vi "Shooter Mode Selector.vi"(9 "Set To Manual?":bool, 10 "Set To Safe?":bool, 11 "Set To Auto?":bool) -> (3 "Mode":T1)   [LabVIEW 2015]
uses:
  Common Code/Shoot Modes Enum.ctl
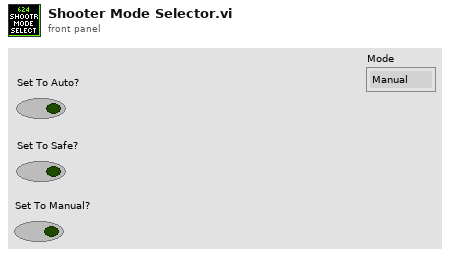
[diagram p1: front panel]
types:
  T1 = typedef "Shoot Modes Enum.ctl" = enum16{"Manual", "Safe", "Auto"}
  T2 = enum16{"0", "1", "2", "3", "4", "5", "6", "7", "8", "9", "A", "B", "C", "D", "E", "F", "G", "H", "I", "J", "K", "L", "M", "N", "O", "P", "Q", "R", "S", "T", "U", "V", "W", "X", "Y", "Z", "F1", "F2", "F3", "F4", "F5", "F6", "F7", "F8", "F9", "F10", "F11", "F12", "F13", "F14", "F15", "ADD", "BACK", "BACKSLASH", "CAPITAL", "COMMA", "DECIMAL", "DELETE", "DIVIDE", "DOWN", "END", "EQUALS", "ESCAPE", "GRAVE (`)", "HOME", "INSERT", "LBRACKET", "LCONTROL", "LEFT", "L ALT", "LSHIFT", "LWIN", "MINUS", "MULTIPLY", "NEXT", "NUMLOCK", "NUMPAD_0", "NUMPAD_1", "NUMPAD_2", "NUMPAD_3", "NUMPAD_4", "NUMPAD_5", "NUMPAD_6", "NUMPAD_7", "NUMPAD_8", "NUMPAD_9", "PAUSE", "PERIOD", "PRIOR (PG UP)", "RBRACKET", "RCONTROL", "RETURN", "RIGHT", "R ALT", "RSHIFT", "RWIN", "SCROLL", "SEMICOLON", "SLASH", "SPACE", "SUBTRACT", "TAB", "UP", "ENTER (num pad)", "' (quote)"}
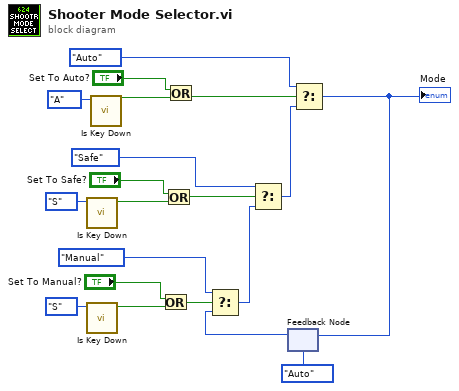
[diagram p0: block diagram]
diagram:
  n1 = call "Is Key Down.vi"("Key"=T2."S") -> ("Key Down?"=w14:bool)  [unwired: 10 in]
  n2 = call "Is Key Down.vi"("Key"=T2."S") -> ("Key Down?"=w10:bool)  [unwired: 10 in]
  n3 = call "Is Key Down.vi"("Key"=T2."A") -> ("Key Down?"=w19:bool)  [unwired: 10 in]
  n4 = Or(x="Set To Manual?", y=w10) -> (x .or. y?=w9:bool)
  n5 = Or(x="Set To Safe?", y=w14) -> (x .or. y?=w13:bool)
  n6 = Or(x="Set To Auto?", y=w19) -> (x .or. y?=w17:bool)
  n7 = feedback #1(Shoot_Modes_Enum."Auto" ("Mode")) -> (w2:T1)
  n8 = Select(t=Shoot_Modes_Enum."Manual" ("Mode"), s=w9, f=w2) -> (s? t:f=w4:T1)
  n9 = Select(t=Shoot_Modes_Enum."Safe" ("Mode"), s=w13, f=w4) -> (s? t:f=w5:T1)
  n10 = Select(t=Shoot_Modes_Enum."Auto" ("Mode"), s=w17, f=w5) -> (s? t:f=w3:T1)
  "Mode" <- w3
  n11 = feedback-in #1(w3) -> ()
